vi "Keep legal squares.vi"(1 "chessboard_size":u8, 2 "squares (chessboard_index)":T1[](array[typedef])) -> (0 "legal squares only (chessboard_index)":T1[](array[typedef]))   [LabVIEW 2020, in "core.lvlib"]
uses:
  core.lvlib
  core_data/chessboard_index.ctl
  core_data/core_data.lvlib
panel:
  out "T = this square is legal\nBoth row and column in range":bool
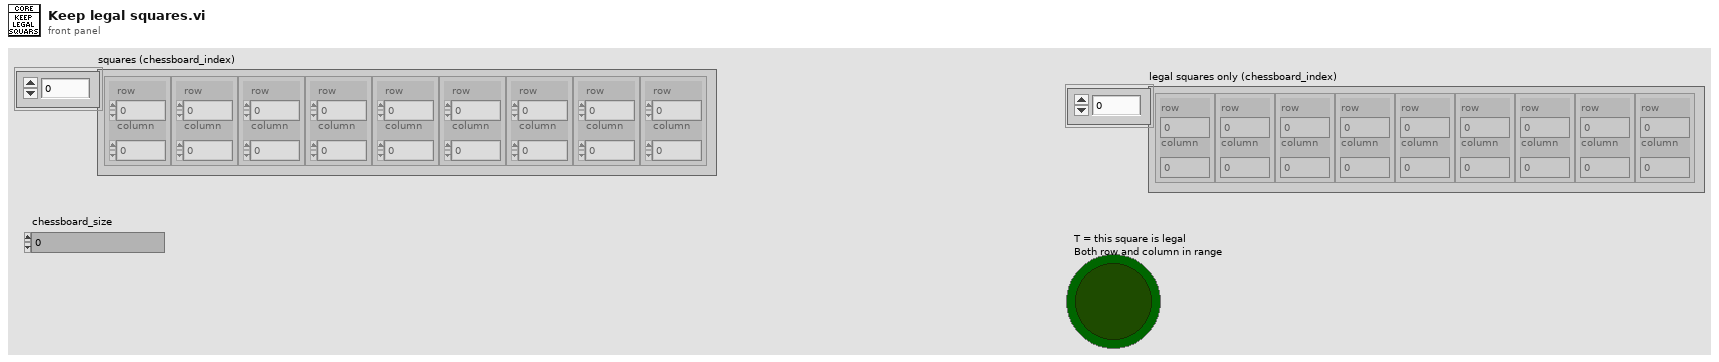
[diagram p1: front panel]
types:
  T1 = typedef "core.lvlib/core_data.lvlib/chessboard_index.ctl" = cluster{"row":u8, "column":u8}
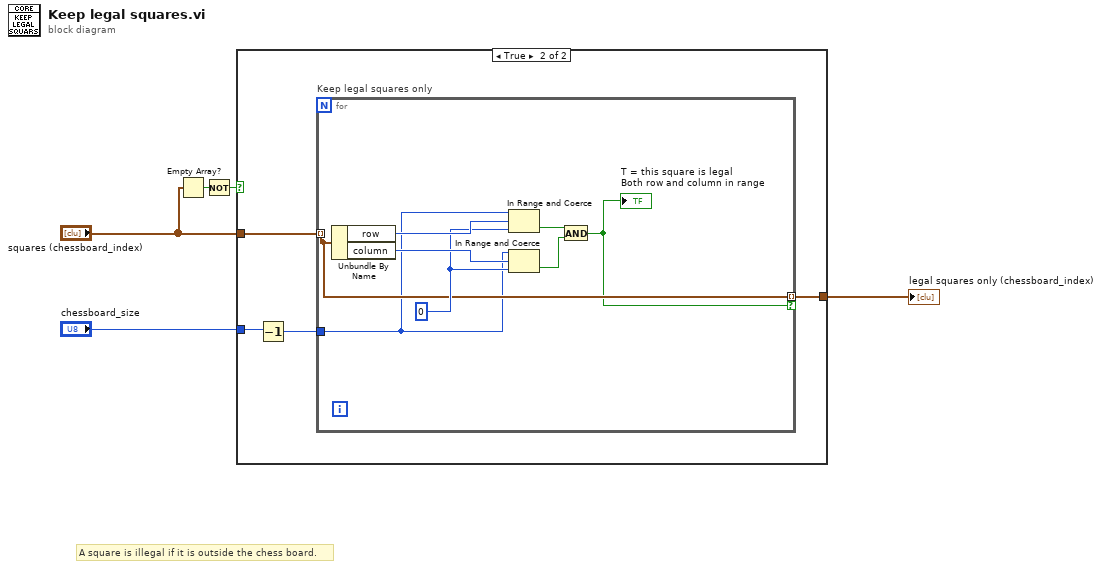
[diagram p0: block diagram]
diagram:
  # "A square is illegal if it is outside the chess board."
  n1 = Empty Array?(array="squares (chessboard_index)") -> (empty?=w3:bool)
  n2 = Not(x=w3) -> (.not. x?=w2:bool)
  n3 = case shown="True" w2 {
    tunnel: "squares (chessboard_index)" -> [_ w9]
    tunnel: [_ w8] -> w5
    tunnel: "chessboard_size" -> [_ w7]
    frame False {
    }
    frame True {
      n4 = Decrement(x=w7) -> (x-1=w6:u8)
      n5 = for "Keep legal squares only" {
        tunnel: w9 -> [w12] mode=indexing
        tunnel: [w12] -> w8 mode=indexing if=w11
        tunnel: w6 -> [w10]
        w14 = u8 0 ("lower limit")
        n6 = Unbundle By Name(w12) -> ("row"=w17:u8, "column"=w15:u8)
        n7 = In Range and Coerce(upper limit=w10, x=w17, lower limit=w14) -> (In Range?=w16:bool)  [unwired: 1 out]
        n8 = In Range and Coerce(upper limit=w10, x=w15, lower limit=w14) -> (In Range?=w13:bool)  [unwired: 1 out]
        n9 = And(x=w16, y=w13) -> (x .and. y?=w11:bool)
        "T = this square is legal\nBoth row and column in range" <- w11
      }
    }
  }
  "legal squares only (chessboard_index)" <- w5
